vi "Waveform Analisys.vi"() -> ()   [LabVIEW 2013]
uses:
  <vilib>/sound2/lvsound2.llb/Sound Data Format.ctl
  <vilib>/sound2/lvsound2.llb/Sampling Mode.ctl
  <vilib>/express/express analysis/Spectral/Block/exnSpectralBlock spectral measurements RMS poly.vi
  <vilib>/express/express analysis/Spectral/Block/exnSpectralBlock spectral measurements RMS WFM.vi
  <vilib>/express/express analysis/Spectral/XNode/ExpressSpectralMeasurementsBlockNode.xnode
  <vilib>/sound2/lvsound2.llb/Sound Input Read (DBL).vi
  <vilib>/measure/NI_MABase.lvlib
  <vilib>/sound2/lvsound2.llb/Sound Output Write (DBL Single).vi
panel:
  in  "Tone":dbl(slide) scale=10.0..100.0
  out "Clean Signal 2":waveform(dbl)(graph)
  in  "data[0]":waveform(dbl)
  in  "number of samples/ch":i32=25000
  out "Distorted Signal":waveform(dbl)(graph)
  in  "Distortion":dbl(slide)=1.0 scale=0.0..1.0
  in  "Gain":dbl(slide)=1.0 scale=0.0..1.0
  in  "stop":bool
  out "Clean Signal":cluster{"f0":dbl, "df":dbl, "magnitude":dbl[]}(graph)
  in  "I/O format":T1={"sample rate (S/s)"=192000.0, "number of channels"=2, "bits per sample"=24}
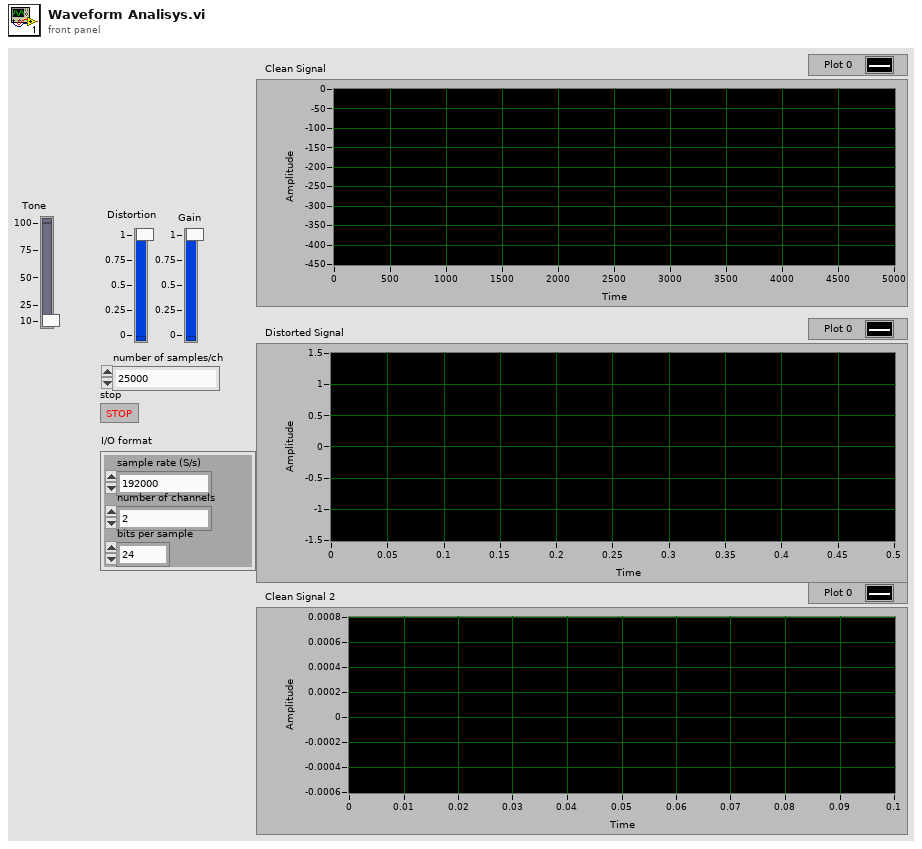
[diagram p1: front panel]
types:
  T1 = typedef "Sound Data Format.ctl" = cluster{"sample rate (S/s)":dbl, "number of channels":i32, "bits per sample":i32}
  T2 = typedef "Sampling Mode.ctl" = i32
  T3 = typedef "Sound Output Task ID.ctl" = u32
  T4 = typedef "Sound Input Task ID.ctl" = u32
  T5 = cluster{"averaging mode":u16, "weighting mode":u16, "number of averages":u32}
  T6 = cluster{"dB On (F)":bool, "unwrap phase (F)":bool, "convert to degree (F)":bool}
  T7 = cluster{"data[0]":waveform(dbl), "data[1]":waveform(dbl), "data[2]":waveform(dbl), "data[3]":waveform(dbl), "data[4]":waveform(dbl), "data[5]":waveform(dbl), "data[6]":waveform(dbl), "data[7]":waveform(dbl), "data[8]":waveform(dbl)}
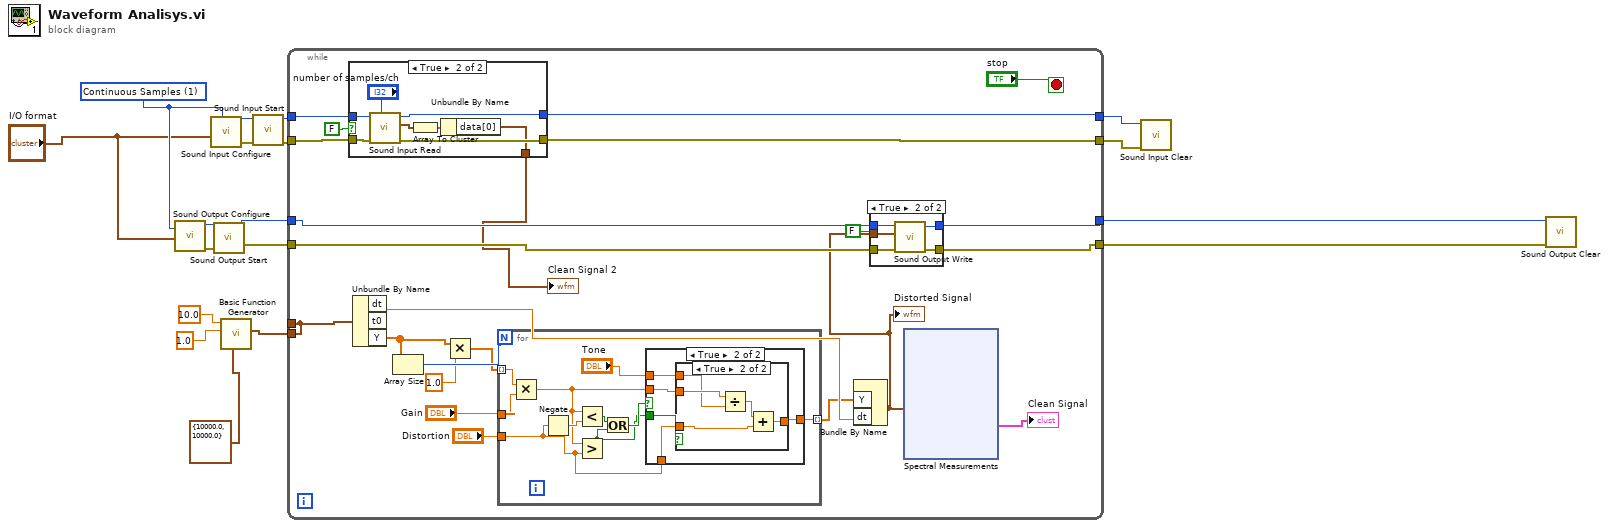
[diagram p0: block diagram]
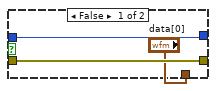
[diagram p3: hidden frame]
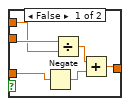
[diagram p5: hidden frame]
diagram:
  w8 = T2 1 items=["Finite Samples", "Continuous Samples"] ("sample mode")
  n1 = call <vilib>:"Sound Output Configure.vi"("sample mode"=w8, "sound format"="I/O format") -> ("error out"=w12:errorcluster, "task ID"=w11:T3)  [unwired: 8 in]
  n2 = call <vilib>:"Sound Input Configure.vi"("sample mode"=w8, "sound format"="I/O format") -> ("error out"=w17:errorcluster, "task ID"=w18:T4)  [unwired: 8 in]
  n3 = call <vilib>:"Sound Output Start.vi"("error in (no error)"=w12, "task ID"=w11) -> ("error out"=w2:errorcluster, "task ID out"=w3:T3)  [unwired: 8 in]
  n4 = call <vilib>:"Basic Function Generator.vi"("sampling info"=cluster{"#s":dbl, "Fs":dbl} {"#s"=10000.0, "Fs"=10000.0}, "amplitude"=1.0, "frequency"=10.0) -> ("signal out"=w1:waveform(dbl))  [unwired: 6 in, 2 out]
  n5 = call <vilib>:"Sound Input Start.vi"("error in (no error)"=w17, "task ID"=w18) -> ("error out"=w15:errorcluster, "task ID out"=w16:T4)  [unwired: 8 in]
  n6 = while {
    tunnel: w16 -> [w41]
    tunnel: w15 -> [w40]
    tunnel: [w39] -> w14
    tunnel: [w38] -> w13
    tunnel: w3 -> [w28]
    tunnel: w2 -> [w30]
    tunnel: [w27] -> w10
    tunnel: [w29] -> w9
    tunnel: [w20] -> _
    tunnel: w1 -> [w20]
    stop <- "stop" stop-if-true
    n7 = case shown="True" FALSE {
      tunnel: w41 -> [w61 w69]
      tunnel: w40 -> [w60 w68]
      tunnel: [w61 w67] -> w39
      tunnel: [w60 w66] -> w38
      tunnel: ["data[0]" w62] -> w19
      frame False {
      }
      frame True {
        n8 = call-poly <vilib>:"Sound Input Read.vi"("number of samples/ch"="number of samples/ch", "error in (no error)"=w68, "task ID"=w69) -> ("error out"=w66:errorcluster, "data"=w63:waveform(dbl)[], "task ID out"=w67:T4)  [unwired: 6 in]
        n9 = Array To Cluster(array=w63) -> (cluster=w65:T7)
        n10 = Unbundle By Name(w65) -> ("data[0]"=w62:waveform(dbl))
      }
    }
    "Clean Signal 2" <- w19
    n11 = Unbundle By Name(w20) -> ("dt"=w33:dbl, "Y"=w23:dbl[])  [unwired: 1 out]
    n12 = Array Size(array=w23) -> (size(s)=w34:i32)
    n13 = Multiply(x=w23, y=1.0) -> (x*y=w22:dbl[])
    n14 = for {
      N: w34 -> [_]
      tunnel: w22 -> [w78] mode=indexing
      tunnel: "Gain" -> [w79]
      tunnel: "Distortion" -> [w76]
      tunnel: [w77] -> w26 mode=indexing
      n15 = Multiply(x=w78, y=w79) -> (x*y=w74:dbl)
      n16 = Negate(x=w76) -> (-x=w75:dbl)
      n17 = Less?(x=w74, y=w75) -> (x < y?=w72:bool)
      n18 = Greater?(x=w74, y=w76) -> (0:w71:bool)
      n19 = Or(x=w72, y=w71) -> (x .or. y?=w73:bool)
      n20 = case shown="True" w73 {
        tunnel: [w80 w82] -> w77
        tunnel: w74 -> [w80 w85]
        tunnel: w76 -> [_ w84]
        tunnel: w71 -> [_ w83]
        tunnel: "Tone" -> [_ w81]
        frame False {
        }
        frame True {
          n21 = case shown="True" w83 {
            tunnel: w85 -> [w87 w93]
            tunnel: w84 -> [w88 w94]
            tunnel: [w90 w95] -> w82
            tunnel: w81 -> [w86 w92]
            frame False {
              n22 = Negate(x=w88) -> (-x=w89:dbl)
              n23 = Divide(x=w87, y=w86) -> (x/y=w91:dbl)
              n24 = Add(x=w91, y=w89) -> (x+y=w90:dbl)
            }
            frame True {
              n25 = Divide(x=w93, y=w92) -> (x/y=w96:dbl)
              n26 = Add(x=w96, y=w94) -> (x+y=w95:dbl)
            }
          }
        }
      }
    }
    n27 = Bundle By Name("Y"=w26, "dt"=w33) -> (w24:waveform(dbl))  [unwired: 1 in]
    "Distorted Signal" <- w24
    n28 = case shown="True" FALSE {
      tunnel: w30 -> [w42 w48]
      tunnel: [w42 w47] -> w29
      tunnel: w28 -> [w43 w46]
      tunnel: [w43 w45] -> w27
      tunnel: w24 -> [_ w44]
      frame False {
      }
      frame True {
        n29 = call-poly <vilib>:"Sound Output Write.vi"("error in (no error)"=w48, "data"=w44, "task ID"=w46) -> ("error out"=w47:errorcluster, "task ID out"=w45:T3)  [unwired: 7 in]
      }
    }
    n30 = xnode "Spectral Measurements"("Signals"=w24) -> ("FFT - (RMS)"=→"Clean Signal":cluster{"f0":dbl, "df":dbl, "magnitude":dbl[]})  [unwired: 1 in, 2 out]
  }
  n31 = call <vilib>:"Sound Input Clear.vi"("error in (no error)"=w13, "task ID"=w14) -> ()  [unwired: 9 in, 1 out]
  n32 = call <vilib>:"Sound Output Clear.vi"("error in (no error)"=w9, "task ID"=w10) -> ()  [unwired: 9 in, 1 out]
